vi "Finalize Turn.vi"(8 "Error in":errorcluster, 10 "Msg Output":refnum<class "Msg Output.lvclass">, 11 "Core Actor in":refnum<class "Core Actor.lvclass">) -> (0 "Error out":errorcluster, 3 "Core Actor out":refnum<class "Core Actor.lvclass">)   [LabVIEW 2025, in "jettl.lvlib" / "Base Actor.lvlib" / "Core Actor.lvclass"]
uses:
  Core Actor.lvclass
  Msg Output/Msg Output.lvclass
  Core Actor.lvclass/Core Actor.ctl
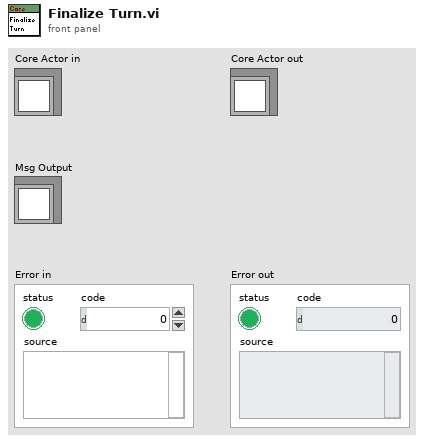
[diagram p1: front panel]
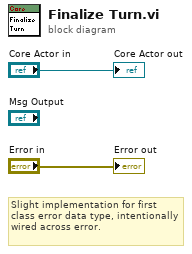
[diagram p0: block diagram]
diagram:
  # "Slight implementation for first class error data type, intentionally wired across error."
  "Core Actor out" <- "Core Actor in"
  "Error out" <- "Error in"
